vi "StopIndex.vi"(0 "Axis In (Axis Space)":T1=enum."Axis Space", 11 "error in (no error)":errorcluster) -> (4 "Axis Out":T1, 15 "error out":errorcluster)   [LabVIEW 2009]
doc: "Stops the currently executing index by disabling the drive and then subsequently re-enabling it. If the drive is not currently executing an index and/or is disabled the function does nothing."
uses:
  typedefs/AxisSelect_Enum.ctl
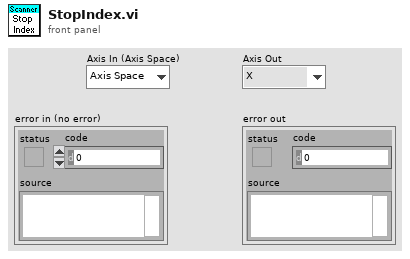
[diagram p1: front panel]
types:
  T1 = typedef "AxisSelect_Enum.ctl" = enum16{"X", "Y", "Z", "Axis Space"}
  T2 = typedef "DriveStatus_Cluster.ctl" = cluster{"In-position":bool, "Zero Speed":bool, "Enabled":bool, "Fault Disable":bool, "Ready":bool, "Start Index":bool, "Overtravel Exceeded":bool, "Up to Speed":bool, "Sequence Complete":bool}
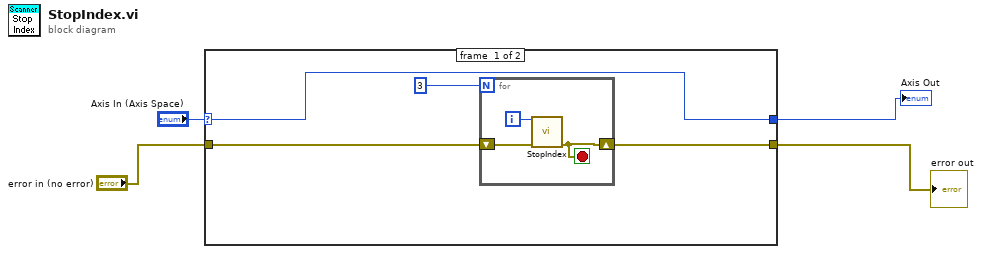
[diagram p0: block diagram]
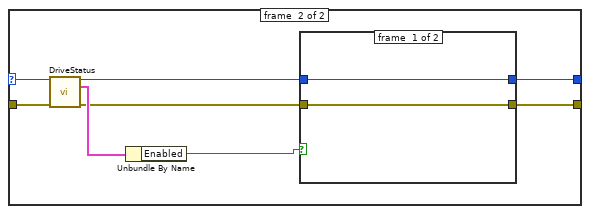
[diagram p2: hidden frame]
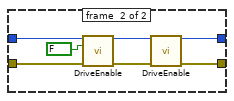
[diagram p3: hidden frame]
diagram:
  n1 = case shown="\"X\"..\"Z\"" "Axis In (Axis Space)" {
    selector: "Axis In (Axis Space)" -> [w7 w17]
    tunnel: [w7 w19] -> w4
    tunnel: [w5 w18] -> w2
    tunnel: "error in (no error)" -> [w6 w13]
    frame #0 {
      n2 = for {
        N: 3 -> [_]
        shift-right: [w9] -> w5
        shift-left: w6 -> [w10]
        i -> [w11]
        stop <- w9 stop-if-true
        n3 = call "StopIndex.vi"("Axis In (Axis Space)"=w11, "error in (no error)"=w10) -> ("error out"=w9:errorcluster)  [unwired: 12 in, 1 out]
      }
    }
    frame #1 {
      n4 = call "DriveStatus.vi"("Axis In"=w17, "error in (no error)"=w13) -> ("Axis Out"=w15:T1, "Status"=w16:T2, "error out"=w14:errorcluster)  [unwired: 11 in]
      n5 = Unbundle By Name(w16) -> ("Enabled"=w12:bool)
      n6 = case shown="True" w12 {
        tunnel: [w20 w27] -> w19
        tunnel: [w21 w26] -> w18
        tunnel: w14 -> [w21 w22]
        tunnel: w15 -> [w20 w28]
        frame #0 {
        }
        frame #1 {
          n7 = call "DriveEnable.vi"("Axis In (Axis Space)"=w28, "Enable (T)"=FALSE, "error in (no error)"=w22) -> ("Axis Out"=w25:T1, "error out"=w24:errorcluster)  [unwired: 11 in]
          n8 = call "DriveEnable.vi"("Axis In (Axis Space)"=w25, "error in (no error)"=w24) -> ("Axis Out"=w27:T1, "error out"=w26:errorcluster)  [unwired: 12 in]
        }
      }
    }
  }
  "Axis Out" <- w4
  "error out" <- w2
